vi "About Phasor Explorer.vi"() -> ()   [LabVIEW 2019]
uses:
  SEPXP Globals.vi
panel:
  in  "OK":bool
  out "Version":string
  out "Phasor  Explorer":string="  Phasor Explorer"
  # "© 2018-2020 The Regents of University of California\nAuthor: X. Michalet, Department of Chemistry & Biochemistry, UCLA\n\nThis software product was developed using LabVIEW™ and the National Instruments Vision Development Toolkit for LabVIEW. Funding was provided in part by grants from the US National Institute of Health (NIH) and the US Department of Energy (DOE).\n\nLabVIEW is a trademark of National Instruments.\nAlliGator is not endorsed by, or sponsored by National Instruments, NIH, DOE or UCLA. This software is provided without guaranty of any kind, whether expressed or implied."
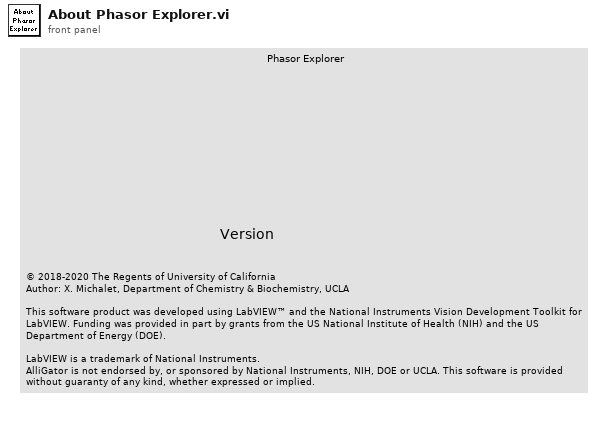
[diagram p1: front panel]
types:
  T1 = enum32{"Invalid", "Standard", "Closed", "Hidden", "Minimized", "Maximized"}
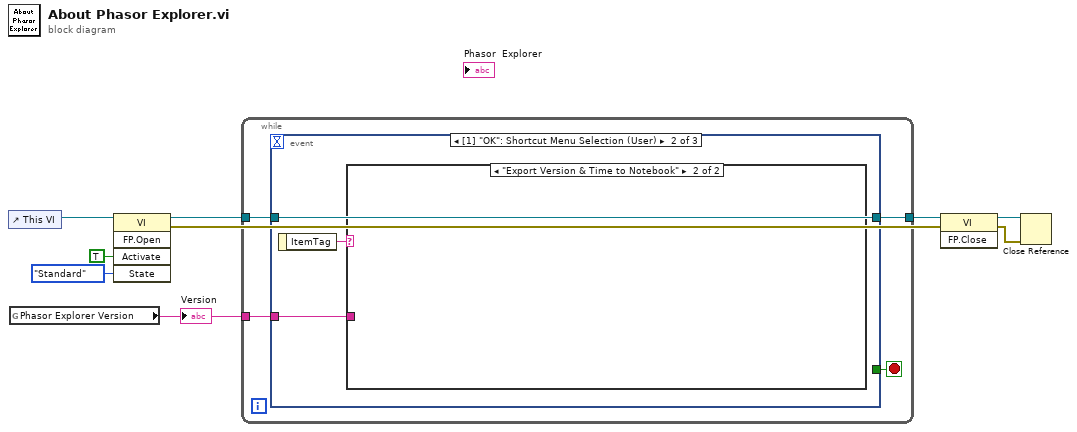
[diagram p0: block diagram]
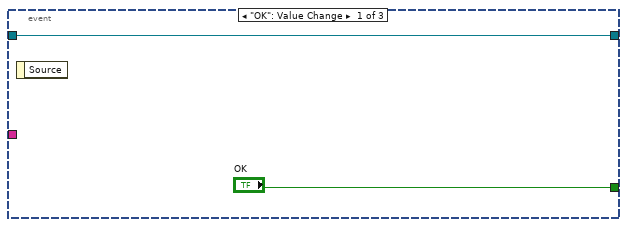
[diagram p2: hidden frame]
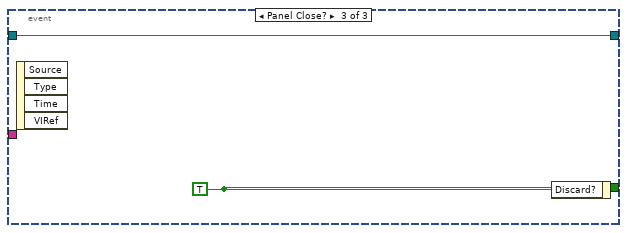
[diagram p4: hidden frame]
diagram:
  n1 = control-ref of="This VI"() -> (w7:refnum<vi>)
  n2 = global read "SEPXP Globals.vi" "Phasor Explorer Version"() -> (w3:string)
  "Version" <- w3
  n3 = invoke class="VI" method="FP.Open"(reference=w7, "Activate"=TRUE ("Activate?"), "State"=T1."Standard") -> (reference out=w6:refnum<vi>, error out=w2:errorcluster)  [unwired: 2 in, 3 out]
  n4 = while {
    tunnel: [w11] -> w9
    tunnel: w6 -> [w12]
    tunnel: w3 -> [w10]
    stop <- w13 stop-if-true
    n5 = event shown="[1] \"OK\": Shortcut Menu Selection (User)" {
      selector: _ -> [_ _ _]
      dyn-events: _ -> [_ _ _]
      timeout: _ -> [_ _ _]
      tunnel: ["OK" _ w20] -> w13
      tunnel: w12 -> [w14 w16 w19]
      tunnel: [w14 w16 w19] -> w11
      tunnel: w10 -> [_ w17 _]
      event "OK": Value Change {
        n6 = event-data() -> ()  [unwired: 1 in, 1 out]
      }
      event "OK": Shortcut Menu Selection (User) {
        n7 = event-data() -> ("ItemTag"=w18:string)  [unwired: 1 in]
        n8 = case shown="\"Export Version & Time to Notebook\"" w18 {
          tunnel: w17 -> [_ _]
          frame "", Default {
          }
          frame "Export Version & Time to Notebook" {
          }
        }
      }
      event Panel Close? {
        w20 = TRUE ("Discard?")
        n9 = event-data() -> ()  [unwired: 1 in, 4 out]
        n10 = event-data("Discard?"=w20) -> ()  [unwired: 1 in, 1 out]
      }
    }
  }
  n11 = invoke class="VI" method="FP.Close"(reference=w9, error in=w2) -> (reference out=w8:refnum<vi>, error out=w1:errorcluster)  [unwired: 1 in, 1 out]
  n12 = Close Reference(reference=w8, error in (no error)=w1) -> ()  [unwired: 1 out]
